vi "LaunchVeriStand.vi"(8 "error in (no error)":errorcluster) -> (0 "error out":errorcluster)   [LabVIEW 2027, in "VeriStandTestUtilities.lvlib"]
uses:
  VeriStandTestUtilities/VeriStandTestUtilities.lvlib
  <vilib>/Utility/sysdir.llb/System Directory Type.ctl
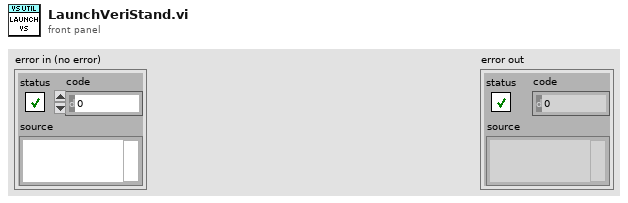
[diagram p1: front panel]
types:
  T1 = typedef "System Directory Type.ctl" = i32
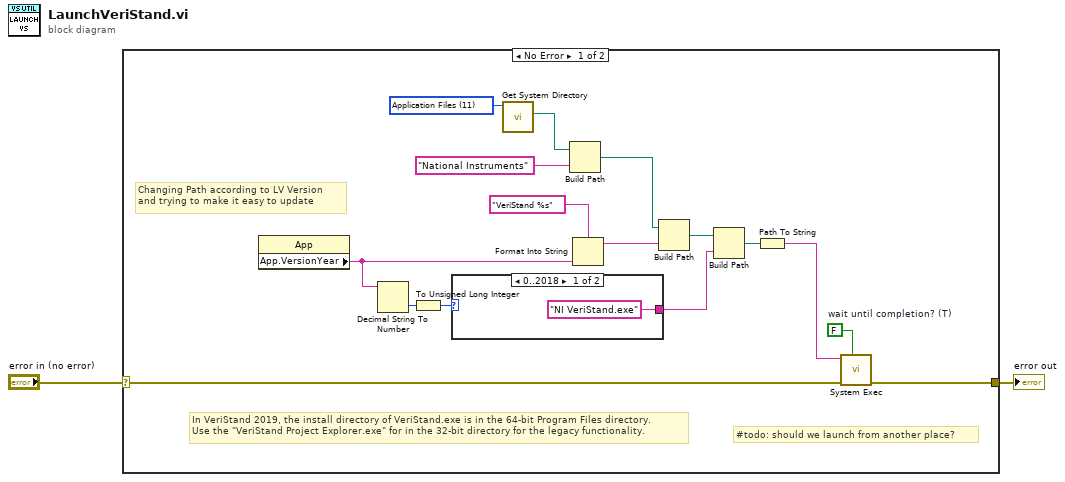
[diagram p0: block diagram]
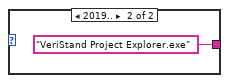
[diagram p2: hidden frame]
diagram:
  n1 = case shown="No Error" "error in (no error)" {
    selector: "error in (no error)" -> [w12 w21]
    tunnel: [w15 w21] -> w1
    frame No Error {
      w11 = T1 11 items=["User Home"=0, "User Desktop"=1, "User Documents"=2, "User Application Data"=3, "User Preferences"=4, "User Temporary"=5, "Public Documents"=6, "Public Application Data"=7, "Public Preferences"=8, "Public Cache"=13, "System Core Libraries"=9, "System Installed Libraries"=10, "Application Files"=11, "Boot Volume Root"=12] ("system directory type")
      w18 = FALSE  # wait until completion? (T)
      # "In VeriStand 2019, the install directory of VeriStand.exe is in the 64-bit Program Files directory.\nUse the \"VeriStand Project Explorer.exe\" for in the 32-bit directory for the legacy functionality."
      # "Changing Path according to LV Version\nand trying to make it easy to update"
      # "#todo: should we launch from another place?"
      n2 = property class="App"() -> ("App.VersionYear"=w13:string)  [unwired: 2 in, 2 out]
      n3 = Decimal String To Number(string=w13) -> (number=w14:i32)  [unwired: 2 in, 1 out]
      n4 = To Unsigned Long Integer(number=w14) -> (unsigned 32bit integer=w3:u32)
      n5 = case shown="0..2018" w3 {
        tunnel: ["NI VeriStand.exe" ("command line") "VeriStand Project Explorer.exe" ("command line")] -> w6
        frame 0..2018 {
        }
        frame 2019.. {
        }
      }
      n6 = call <vilib>:"Get System Directory.vi"("system directory type"=w11) -> ("system directory"=w9:path)  [unwired: 10 in]
      n7 = Build Path(base path=w9, name or relative path="National Instruments" ("command line")) -> (appended path=w8:path)
      n8 = Format Into String(format string="VeriStand %s" ("command line"), w13) -> (resulting string=w7:string)  [unwired: 2 in, 1 out]
      n9 = Build Path(base path=w8, name or relative path=w7) -> (appended path=w5:path)
      n10 = Build Path(base path=w5, name or relative path=w6) -> (appended path=w16:path)
      n11 = Path To String(path=w16) -> (string=w17:string)
      n12 = call <vilib>:"System Exec.vi"("wait until completion? (T)"=w18, "error in (no error)"=w12, "command line"=w17) -> ("error out"=w15:errorcluster)  [unwired: 5 in, 3 out]
    }
    frame Error {
    }
  }
  "error out" <- w1
